vi "Read and Update Key.vi"   [LabVIEW 2016, in "_Configurations.lvlib" / "Configurations.lvclass"]
uses:
  Configurations.lvclass
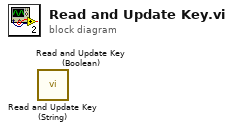
[diagram p0: block diagram]
diagram:
  n1 = call "Read and Update Key (String).vi"() -> ()  [unwired: 13 in, 3 out]
  n2 = call "Read and Update Key (Boolean).vi"() -> ()  [unwired: 13 in, 3 out]
